vi "project.vi"() -> ()   [LabVIEW 2017]
uses:
  <vilib>/vision/NI_Vision_Development_Module.lvlib
panel:
  out "min count of cancer\n affected cells":dbl
  out "WBC Count in ml":dbl
  in  "OK Button":bool
  out "error out 5":errorcluster
  in  "Image Pixels (U16)":u16[][](array[numeric])
  out "neagative image 3":T1(plugin-control)
  out "edge detection 2":T1(plugin-control)
  out "error out 4":errorcluster
  out "error out 3":errorcluster
  out "threhsold image":T1(plugin-control)
  in  "Image Type 2":T2 items=["Grayscale (U8)", "Grayscale (I16)", "Grayscale (SGL)", "Complex (CSG)", "RGB (U32)", "HSL (U32)", "RGB (U64)", "Grayscale (U16)"]
  in  "Border Size":i32=3
  in  "Image Type":T2 items=["Grayscale (U8)", "Grayscale (I16)", "Grayscale (SGL)", "Complex (CSG)", "RGB (U32)", "HSL (U32)", "RGB (U64)", "Grayscale (U16)"]
  out "error out":errorcluster
  out "Image":T1(plugin-control)
  in  "File Path":path
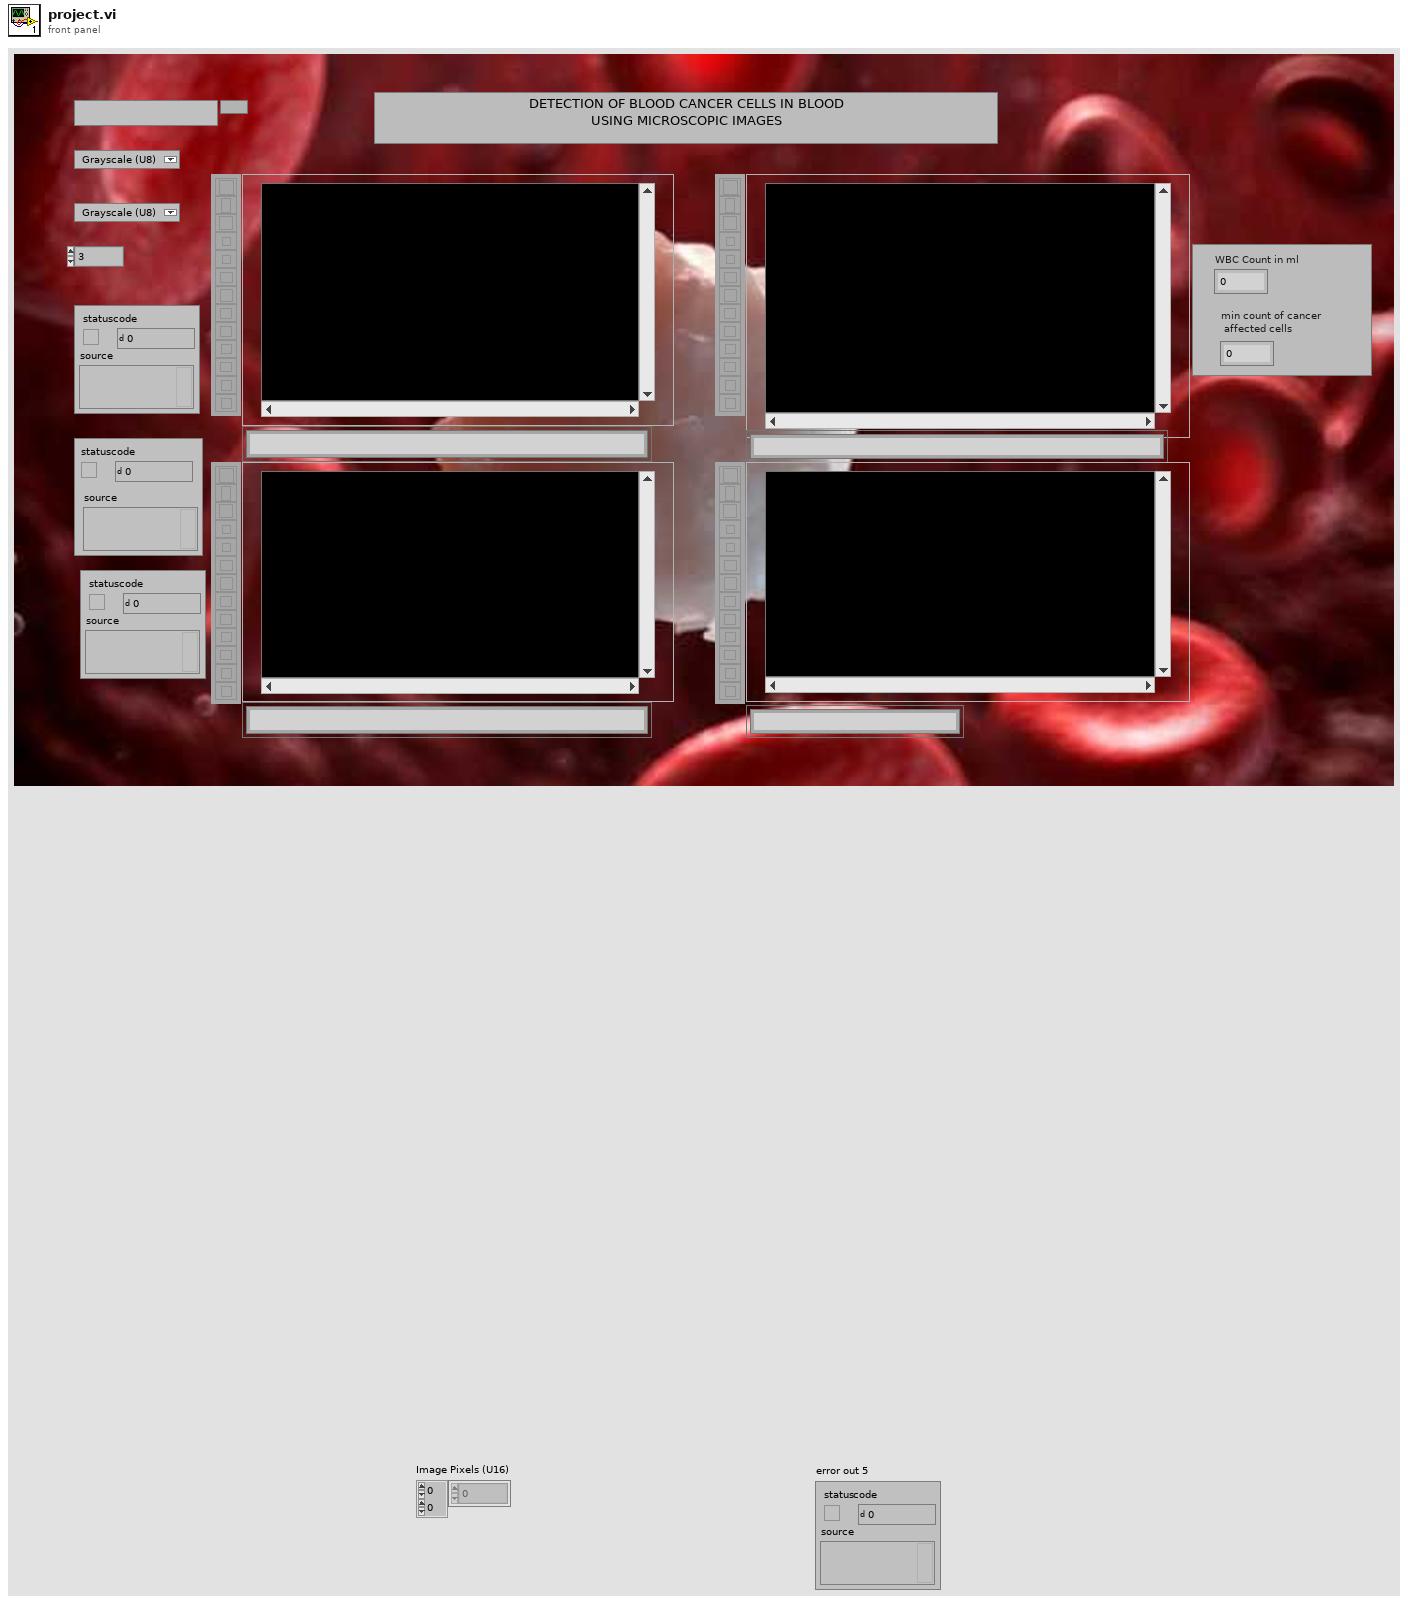
[diagram p1: front panel]
types:
  T1 = typedef "IMAQ Image.ctl" = refnum<image>
  T2 = typedef "Image Type" = u32
  T3 = cluster{"Lower value":sgl, "Upper value":sgl, "Replace Value":sgl, "Keep/Replace Value (Replace)":bool}[]
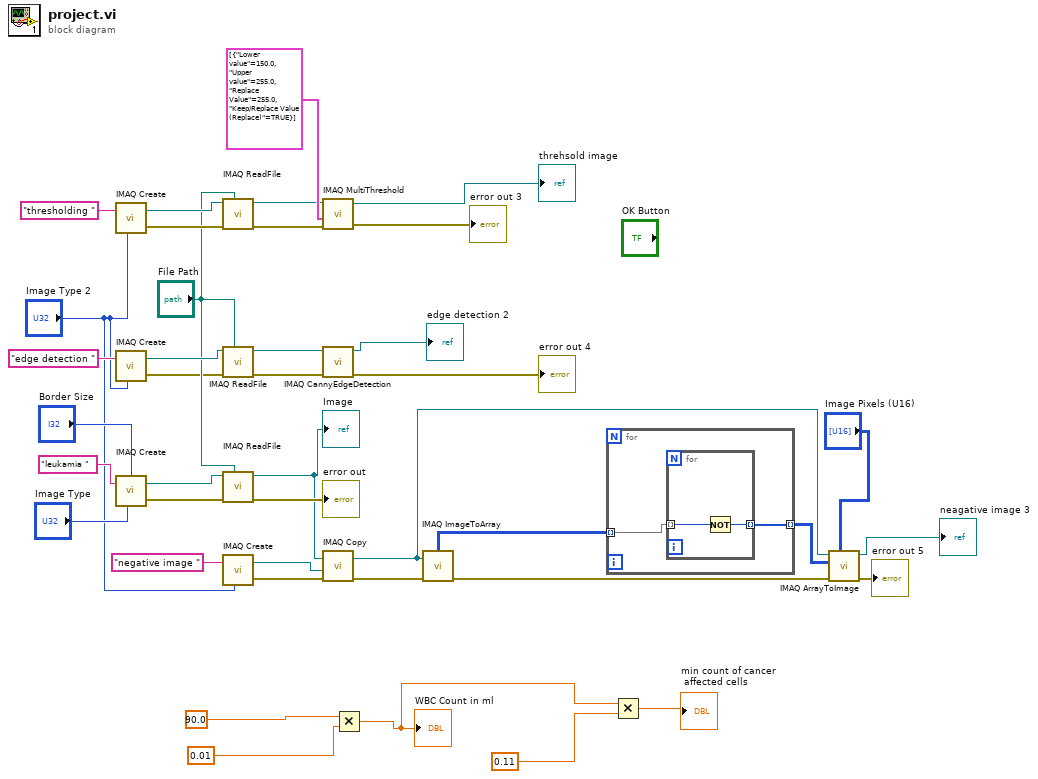
[diagram p0: block diagram]
diagram:
  n1 = call "IMAQ Create"("Image Name"="thresholding ", "Image Type"="Image Type 2") -> ("New Image"=w33:T1, "error out"=w32:errorcluster)  [unwired: 3 in]
  n2 = call "IMAQ Create"("Image Name"="edge detection ", "Image Type"="Image Type 2") -> ("New Image"=w28:T1, "error out"=w23:errorcluster)  [unwired: 3 in]
  n3 = call "IMAQ Create"("Border Size"="Border Size", "Image Name"="leukamia ", "Image Type"="Image Type") -> ("New Image"=w39:T1, "error out"=w37:errorcluster)  [unwired: 2 in]
  n4 = call "IMAQ ReadFile"("File Path"="File Path", "error in (no error)"=w32, "Image"=w33) -> ("error out"=w31:errorcluster, "Image Out"=w21:T1)  [unwired: 4 in, 3 out]
  n5 = call "IMAQ ReadFile"("File Path"="File Path", "error in (no error)"=w23, "Image"=w28) -> ("error out"=w22:errorcluster, "Image Out"=w26:T1)  [unwired: 4 in, 3 out]
  n6 = call "IMAQ ReadFile"("File Path"="File Path", "error in (no error)"=w37, "Image"=w39) -> ("error out"=→"error out":errorcluster, "Image Out"=w6:T1)  [unwired: 4 in, 3 out]
  "Image" <- w6
  n7 = call "IMAQ Create"("Image Name"="negative image ", "Image Type"="Image Type 2") -> ("New Image"=w19:T1, "error out"=w20:errorcluster)  [unwired: 3 in]
  n8 = call "IMAQ MultiThreshold"("error in (no error)"=w31, "Threshold Data"=T3 [{"Lower value"=150.0, "Upper value"=255.0, "Replace Value"=255.0, "Keep/Replace Value (Replace)"=TRUE}], "Image Src"=w21) -> ("error out"=→"error out 3":errorcluster, "Image Dst Out"=→"threhsold image":T1)  [unwired: 2 in]
  n9 = call "IMAQ CannyEdgeDetection"("Image Src"=w26, "error in (no error)"=w22) -> ("Image Dst Out"=→"edge detection 2":T1, "error out"=→"error out 4":errorcluster)  [unwired: 6 in]
  n10 = call "IMAQ Copy"("error in (no error)"=w20, "Image Dst"=w19, "Image Src"=w6) -> ("error out"=w18:errorcluster, "Image Dst Out"=w14:T1)  [unwired: 3 in]
  n11 = Multiply(x=90.0, y=0.01) -> (x*y=w3:dbl)
  "WBC Count in ml" <- w3
  n12 = call "IMAQ ImageToArray"("error in (no error)"=w18, "Image"=w14) -> ("error out"=w15:errorcluster, "Image Pixels (U8)"=w12:u8[][])  [unwired: 2 in, 3 out]
  n13 = for {
    tunnel: w12 -> [w42] mode=indexing
    tunnel: [w41] -> w17 mode=indexing
    n14 = for {
      tunnel: w42 -> [w44] mode=indexing
      tunnel: [w43] -> w41 mode=indexing
      n15 = Not(x=w44) -> (.not. x?=w43:u8)
    }
  }
  n16 = Multiply(x=w3, y=0.11) -> (x*y=→"min count of cancer\n affected cells":dbl)
  n17 = call "IMAQ ArrayToImage"("Image Pixels (U16)"="Image Pixels (U16)", "error in (no error)"=w15, "Image Pixels (U8)"=w17, "Image"=w14) -> ("error out"=→"error out 5":errorcluster, "Image Out"=→"neagative image 3":T1)  [unwired: 6 in]
